vi "set memory.vi"(8 "error in (no error)":errorcluster caption="에러 입력(에러 없음)", 10 "WF List":T1[](array[typedef]), 11 "DW7802 입력":refnum<class "DW7802.lvclass">) -> (0 "error out":errorcluster caption="에러 출력", 3 "DW7802 출력":refnum<class "DW7802.lvclass">)   [LabVIEW 2020, in "DW7802.lvclass"]
uses:
  DW7802.lvclass
  SubVIs/Waveform Editor/Controls/(Ctrl)Waveform Editor_WF List.ctl
  Waveform Obj Class/Waveform Obj/Waveform Obj.lvclass
  Haptic IC/Haptic IC.lvclass/Haptic IC.ctl
  SubVIs/I2C/Instance VIs/(SubVI)I2C_8Bit-8Bit_Write_Single.vi
  SubVIs/I2C/Instance VIs/(SubVI)I2C_8Bit-8Bit_Write_Sequential.vi
  DW7802.lvclass/DW7802.ctl
  Haptic IC/Haptic IC.lvclass
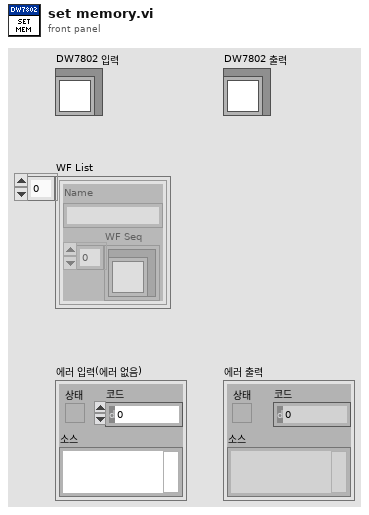
[diagram p1: front panel]
types:
  T1 = typedef "(Ctrl)Waveform Editor_WF List.ctl" = cluster{"Name":string, "WF Seq":refnum<class "Waveform Obj.lvclass">[]}
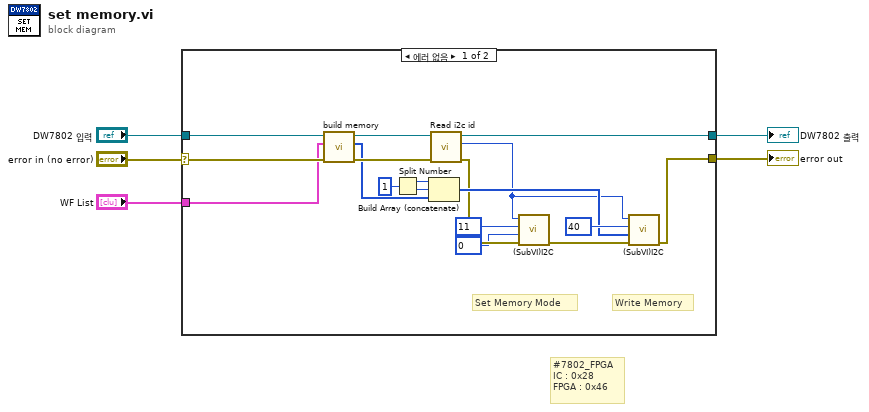
[diagram p0: block diagram]
diagram:
  # "#7802_FPGA\nIC : 0x28\nFPGA : 0x46"
  n1 = case shown="에러 없음" "error in (no error)" {
    selector: "error in (no error)" -> [w16 w25]
    tunnel: [w17 w25] -> w5
    tunnel: "DW7802 입력" -> [w14 w24]
    tunnel: [w23 w24] -> w4
    tunnel: "WF List" -> [w12 _]
    frame No Error {
      # "Write Memory"
      # "Set Memory Mode"
      n2 = call-dynamic "build memory.vi"("error in (no error)"=w16, "WF List"=w12, "DW7802 입력"=w14) -> ("error out"=w15:errorcluster, "full memory data"=w11:u8[], "DW7802 출력"=w13:refnum<class "DW7802.lvclass">)  [unwired: 5 in, 1 out]
      n3 = Split Number(x=u16 1) -> (hi(x)=w20:u8, lo(x)=w19:u8)
      n4 = Build Array (concatenate)(w20, w19, w11) -> (w18:u8[])
      n5 = call "Read i2c id.vi"("error in (no error)"=w15, "Haptic IC 입력"=w13) -> ("error out"=w7:errorcluster, "i2c id"=w8:u8, "Haptic IC 출력"=w23:refnum<class "DW7802.lvclass">)  [unwired: 7 in]
      n6 = call-poly "(SubVI)I2C.vi"("error in (no error)"=w7, "Data to Write"=u8 0, "Address"=u8 11, "ID"=w8) -> ("error out"=w9:errorcluster)  [unwired: 6 in, 1 out]
      n7 = call-poly "(SubVI)I2C.vi"("error in (no error)"=w9, "Data to Write"=w18, "Start Address"=u8 40, "ID"=w8) -> ("error out"=w17:errorcluster)  [unwired: 6 in, 1 out]
    }
    frame Error {
    }
  }
  "error out" <- w5
  "DW7802 출력" <- w4
